vi "Write Stunt.vi"(8 "error in":errorcluster, 10 "Array In":i32[][](array[numeric]), 11 "file path (empty creates file in temp folder)":path) -> (0 "error out":errorcluster)   [LabVIEW 2019, in "flashcards.lvlib"]
uses:
  flashcards.lvlib
  Colors.ctl
panel:
  in  "Colors":T1=enum."White"
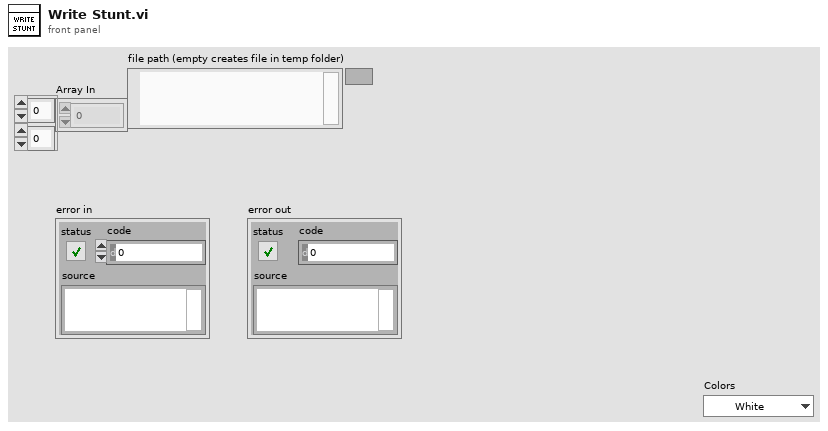
[diagram p1: front panel]
types:
  T1 = typedef "flashcards.lvlib/Colors.ctl" = enum16{"Black", "White", "Orange", "Red", "Blue", "Green", "None"}
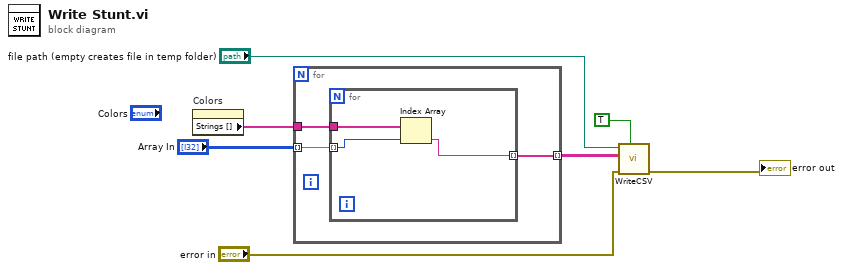
[diagram p0: block diagram]
diagram:
  n1 = property on="Colors" class="Enum (strict)"() -> ("Strings []"=w2:string[])  [unwired: 2 in, 2 out]
  n2 = for {
    tunnel: "Array In" -> [w10] mode=indexing
    tunnel: [w9] -> w5 mode=indexing
    tunnel: w2 -> [w8]
    n3 = for {
      tunnel: w10 -> [w12] mode=indexing
      tunnel: [w11] -> w9 mode=indexing
      tunnel: w8 -> [w13]
      n4 = Index Array(array=w13, index=w12) -> (element=w11:string)
    }
  }
  n5 = call "WriteCSV.vi"("Overwrite File if Exists? (F - append suffix)"=TRUE, "error in (no error)"="error in", "Data to Write"=w5, "file path (empty creates file in temp folder)"="file path (empty creates file in temp folder)") -> ("error out"=→"error out":errorcluster)  [unwired: 6 in, 1 out]
